vi "ReadArrayFromFile.vi"() -> (3 "Output":dbl[](array[numeric]))   [LabVIEW 2018]
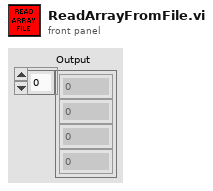
[diagram p1: front panel]
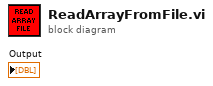
[diagram p0: block diagram]
diagram:
